vi "Finalize Data.vi"(8 "error in (no error)":errorcluster, 11 "Core Threads Configuration in":refnum<class "Core Threads Configuration.lvclass">) -> (0 "error out":errorcluster, 1 "data version":T1, 2 "data":string, 3 "Core Threads Configuration out":refnum<class "Core Threads Configuration.lvclass">)   [LabVIEW 2017, in "DSF Core.lvlib" / "Core Threads Configuration.lvclass"]
uses:
  Core Threads Configuration.lvclass
  C:/Git/DSF/Core/Classes/Configuration/Configuration.lvclass
  Typedefs/DSF Version Info.ctl
  Core Threads Configuration.lvclass/Core Threads Configuration.ctl
  Configuration.lvclass
  DSF Core.lvlib
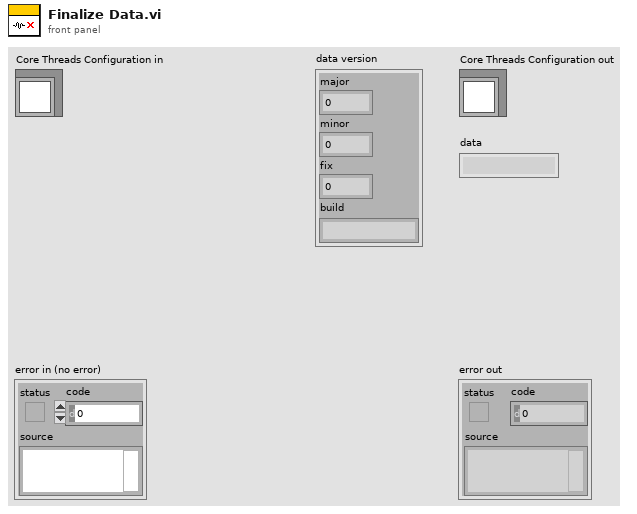
[diagram p1: front panel]
types:
  T1 = typedef "DSF Core.lvlib/DSF Version Info.ctl" = cluster{"major":u32, "minor":u32, "fix":u32, "build":string}
  T2 = typedef "DSF Core.lvlib/DSF Core Thread Configuration.ctl" = cluster{"processor":i32, "priority offset":i16}
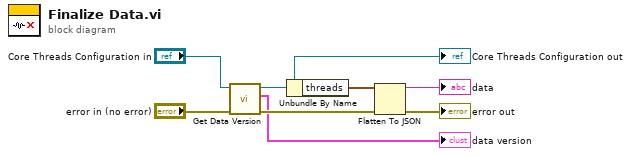
[diagram p0: block diagram]
diagram:
  n1 = call "Get Data Version.vi"("error in (no error)"="error in (no error)", "Configuration in"="Core Threads Configuration in") -> ("error out"=w3:errorcluster, "data version"=→"data version":T1, "Configuration out"=w4:refnum<class "Core Threads Configuration.lvclass">)  [unwired: 7 in]
  "Core Threads Configuration out" <- w4
  n2 = Unbundle By Name(w4) -> ("threads"=w8:T2[])
  n3 = Flatten To JSON(anything=w8, error in (no error)=w3) -> (JSON string=→"data":string, 11:→"error out":errorcluster)  [unwired: 1 in]
